vi "API.vi"(8 "error in (no error)":errorcluster, 11 "AbortManager in":refnum<class "AbortManager.lvclass">) -> (0 "error out":errorcluster, 2 "API":refnum<class "API.lvclass">, 3 "AbortManager out":refnum<class "AbortManager.lvclass">)   [LabVIEW 2020, in "Volatus.lvlib" / "AbortManager.lvclass"]
uses:
  AbortManager.lvclass
  API/API.lvclass
  <vilib>/ActorFramework/Message Enqueuer/Init from Existing Queue.vi
  <vilib>/ActorFramework/Message Enqueuer/Message Enqueuer.lvclass
  <vilib>/ActorFramework/Actor/Actor.lvclass
  C:/Program Files (x86)/National Instruments/LabVIEW 2020/vi.lib/ActorFramework/Actor/Actor.lvclass
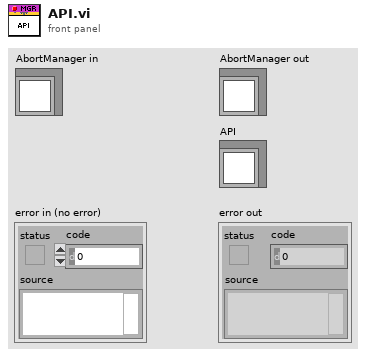
[diagram p1: front panel]
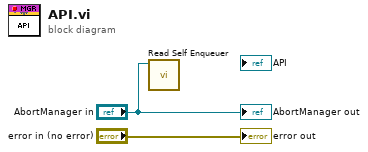
[diagram p0: block diagram]
diagram:
  n1 = call <vilib>:"Read Self Enqueuer.vi"("Actor"="AbortManager in") -> ()  [unwired: 10 in, 1 out]
  "error out" <- "error in (no error)"
  "AbortManager out" <- "AbortManager in"
